vi "Style_Container.vi"() -> ()   [LabVIEW 2025]
panel:
  out "Boolean":bool
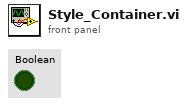
[diagram p1: front panel]
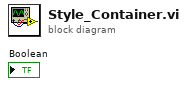
[diagram p0: block diagram]
diagram:
